vi "SLT Get Process Memory Info.vi"(0 "handle":i64, 11 "error in (no error)":errorcluster) -> (4 "handle out":i64, 6 "Physical Usage":u64, 8 "Virtual Usage":u64, 15 "error out":errorcluster)   [LabVIEW 2013, in "ProcessInfo.lvlib"]
uses:
  ProcessInfo.lvlib
  psapi.dll
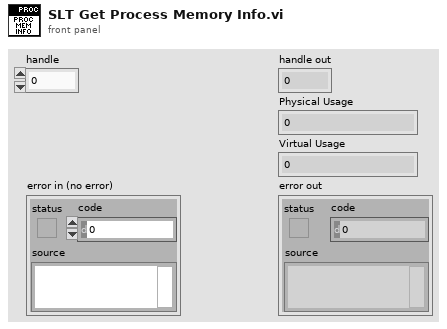
[diagram p1: front panel]
types:
  T1 = cluster{"cb":u32, "PageFaultCount":u32, "PeakWorkingSetSize":u32, "WorkingSetSize":u32, "QuotaPeakPagedPoolUsage":u32, "QuotaPagedPoolUsage":u32, "QuotaPeakNonPagedPoolUsage":u32, "QuotaNonPagedPoolUsage":u32, "PagefileUsage":u32, "PeakPagefileUsage":u32}
  T2 = cluster{"cb":u64, "PageFaultCount":u64, "PeakWorkingSetSize":u64, "WorkingSetSize":u64, "QuotaPeakPagedPoolUsage":u64, "QuotaPagedPoolUsage":u64, "QuotaPeakNonPagedPoolUsage":u64, "QuotaNonPagedPoolUsage":u64, "PagefileUsage":u64, "PeakPagefileUsage":u64}
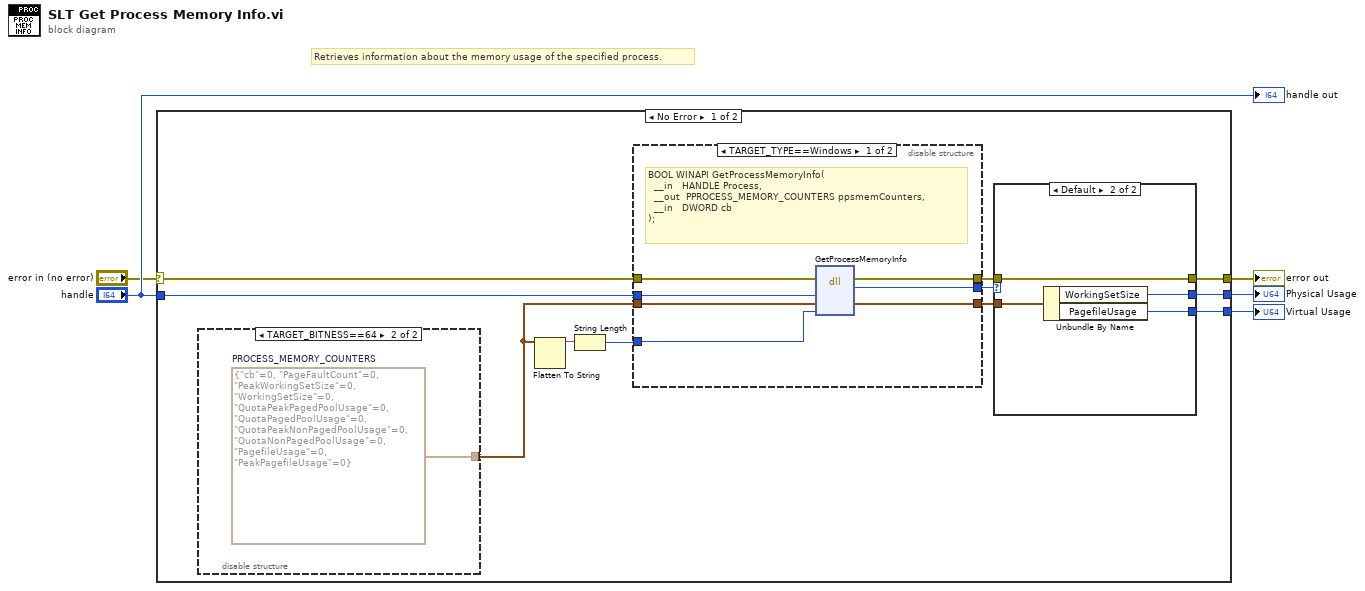
[diagram p0: block diagram]
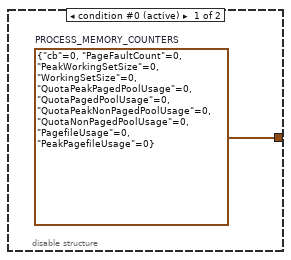
[diagram p3: hidden frame]
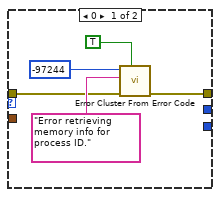
[diagram p4: hidden frame]
diagram:
  # "Retrieves information about the memory usage of the specified process."
  n1 = case shown="No Error" "error in (no error)" {
    selector: "error in (no error)" -> [w15 w38]
    tunnel: [w14 w38] -> w1
    tunnel: "handle" -> [w16 _]
    tunnel: [w13 _] -> w4
    tunnel: [w12 _] -> w5
    frame No Error {
      n2 = disable-structure shown="TARGET_BITNESS==64" {
        disable-tunnel: [w27 w28] -> w10
        frame condition #0 (active) {
          w27 = T1 {"cb"=0, "PageFaultCount"=0, "PeakWorkingSetSize"=0, "WorkingSetSize"=0, "QuotaPeakPagedPoolUsage"=0, "QuotaPagedPoolUsage"=0, "QuotaPeakNonPagedPoolUsage"=0, "QuotaNonPagedPoolUsage"=0, "PagefileUsage"=0, "PeakPagefileUsage"=0}  # PROCESS_MEMORY_COUNTERS
        }
        frame condition #1 {
          w28 = T2 {"cb"=0, "PageFaultCount"=0, "PeakWorkingSetSize"=0, "WorkingSetSize"=0, "QuotaPeakPagedPoolUsage"=0, "QuotaPagedPoolUsage"=0, "QuotaPeakNonPagedPoolUsage"=0, "QuotaNonPagedPoolUsage"=0, "PagefileUsage"=0, "PeakPagefileUsage"=0}  # PROCESS_MEMORY_COUNTERS
        }
      }
      n3 = Flatten To String(anything=w10) -> (data string=w11:string)  [unwired: 1 in, 4 out]
      n4 = String Length(string=w11) -> (length=w9:i32)
      n5 = disable-structure shown="TARGET_TYPE==Windows" {
        disable-tunnel: w16 -> [w23 w25]
        disable-tunnel: w15 -> [w22 w26]
        disable-tunnel: w10 -> [w21 w24]
        disable-tunnel: w9 -> [w20 _]
        disable-tunnel: [w19 w25] -> w8
        disable-tunnel: [w18 w26] -> w7
        disable-tunnel: [w17 w24] -> w6
        frame condition #0 (active) {
          # "BOOL WINAPI GetProcessMemoryInfo(\n  __in   HANDLE Process,\n  __out  PPROCESS_MEMORY_COUNTERS ppsmemCounters,\n  __in   DWORD cb\n);"
          n6 = dll-call lib="psapi.dll" fn="GetProcessMemoryInfo"(error in=w22, "handle"=w23, "PROCESS_MEMORY_COUNTERS"=w21, "cb"=w20) -> (error out=w18:errorcluster, "error"=w19:i32, "PROCESS_MEMORY_COUNTERS"=w17:T1)  [unwired: 4 in, 1 out]
        }
        frame condition #1 {
        }
      }
      n7 = case shown="Default" w8 {
        tunnel: w7 -> [w30 w37]
        tunnel: [w29 w37] -> w14
        tunnel: w6 -> [_ w36]
        tunnel: [_ w35] -> w13
        tunnel: [_ w34] -> w12
        frame 0 {
          n8 = call <vilib>:"Error Cluster From Error Code.vi"("show call chain? (False)"=TRUE, "error in (no error)"=w30, "error message (\"\")"="Error retrieving memory info for  process ID." ("error message (\"\")"), "error code (0)"=-97244) -> ("error out"=w29:errorcluster)  [unwired: 5 in]
        }
        frame Default {
          n9 = Unbundle By Name(w36) -> ("WorkingSetSize"=w35:u32, "PagefileUsage"=w34:u32)
        }
      }
    }
    frame Error {
    }
  }
  "error out" <- w1
  "Physical Usage" <- w4
  "Virtual Usage" <- w5
  "handle out" <- "handle"
